vi "Determine Center of Gravity.vi"(0 "Input Intersections":T1(array[cluster])) -> (1 "CenterOfGravity X":dbl, 2 "CenterOfGravity Y":dbl)   [LabVIEW 2014, in "Position.lvclass"]
uses:
  Position.lvclass
  <vilib>/Analysis/NI_AALBase.lvlib
panel:
  out "y no":i32
  out "x no":i32
  out "x no":i32
  out "y no":i32
  # "This VI determines the center of gravity from a surface area.\nNotation: (x, y)"
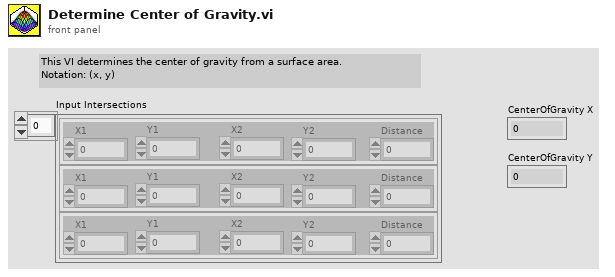
[diagram p1: front panel]
types:
  T1 = cluster{"X1":dbl, "Y1":dbl, "X2":dbl, "Y2":dbl, "Distance":dbl}[]
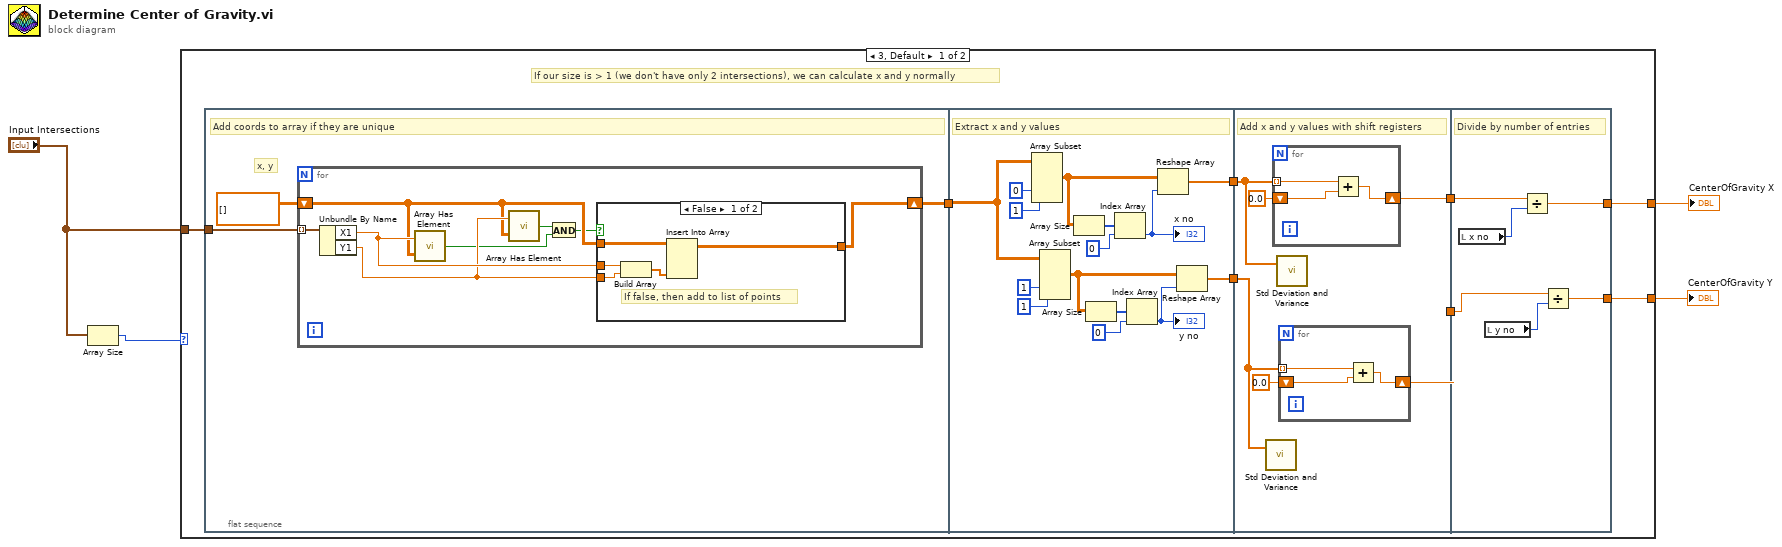
[diagram p0: block diagram]
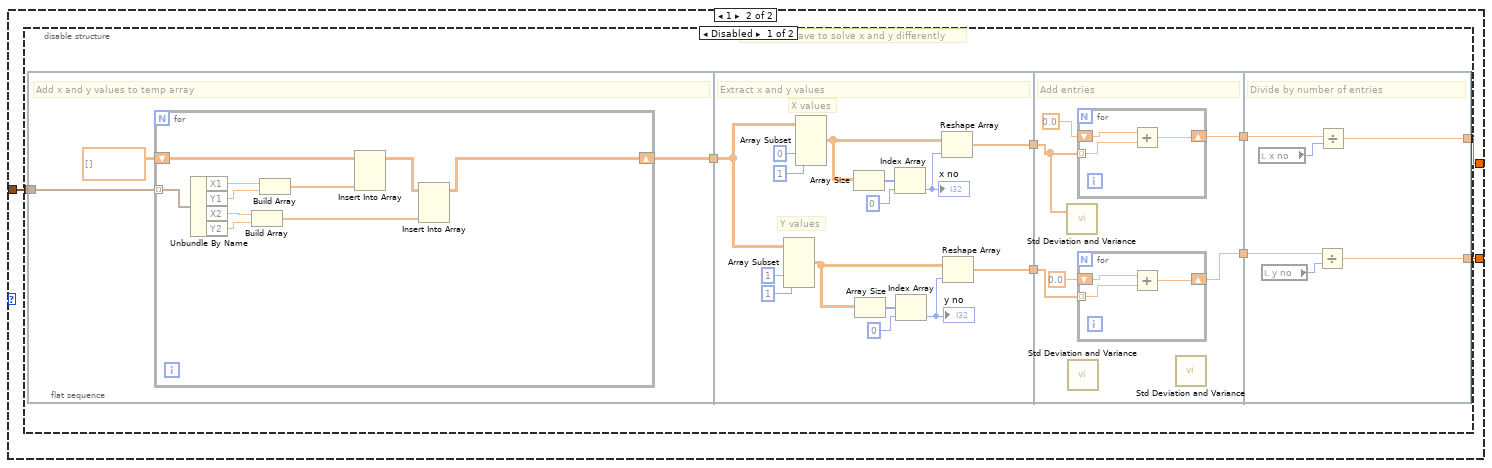
[diagram p3: hidden frame]
diagram:
  n1 = Array Size(array="Input Intersections") -> (size(s)=w1:i32)
  n2 = case shown="3, Default" w1 {
    tunnel: "Input Intersections" -> [w7 w65]
    tunnel: [w6 w63] -> w3
    tunnel: [w5 w64] -> w2
    frame 3, Default {
      # "If our size is > 1 (we don't have only 2 intersections), we can calculate x and y normally"
      n3 = flat-sequence {
        tunnel: w7 -> [w15]
        tunnel: [w14] -> w12
        tunnel: [w40] -> w11
        tunnel: [w39] -> w10
        tunnel: w12 -> [w30]
        tunnel: w11 -> [w46]
        tunnel: w10 -> [w45]
        tunnel: [w48] -> w9
        tunnel: [w47] -> w8
        tunnel: w9 -> [w61]
        tunnel: w8 -> [w60]
        tunnel: [w58] -> w6
        tunnel: [w57] -> w5
        frame #0 {
          # "x, y"
          # "Add coords to array if they are unique"
          n4 = for {
            tunnel: w15 -> [w23] mode=indexing
            shift-right: [w22] -> w14
            shift-left: dbl[][] [] -> [w19]
            n5 = Unbundle By Name(w23) -> ("X1"=w21:dbl, "Y1"=w20:dbl)
            n6 = call "Array Has Element.vi"("Array"=w19, "Element"=w21) -> ("Array has element?"=w17:bool)
            n7 = call "Array Has Element.vi"("Array"=w19, "Element"=w20) -> ("Array has element?"=w18:bool)
            n8 = And(x=w18, y=w17) -> (x .and. y?=w16:bool)
            n9 = case shown="False" w16 {
              tunnel: w21 -> [w27 _]
              tunnel: w20 -> [w26 _]
              tunnel: w19 -> [w28 w29]
              tunnel: [w24 w29] -> w22
              frame False {
                # "If false, then add to list of points"
                n10 = Build Array(w27, w26) -> (w25:dbl[])
                n11 = Insert Into Array(array=w28, new element=w25) -> (w24:dbl[][])  [unwired: 2 in]
              }
              frame True {
                # "If true, then don't add to list of points"
              }
            }
          }
        }
        frame #1 {
          # "Extract x and y values"
          n12 = Array Subset(array=w30, index (col)=0 ("index"), length (col)=1 ("length")) -> (w34:dbl[][])  [unwired: 2 in]
          n13 = Array Subset(array=w30, index (col)=1 ("index"), length (col)=1 ("length")) -> (w38:dbl[][])  [unwired: 2 in]
          n14 = Array Size(array=w34) -> (size(s)=w33:i32[])
          n15 = Array Size(array=w38) -> (size(s)=w37:i32[])
          n16 = Index Array(array=w33, index=0) -> (element=w31:i32)
          "x no" <- w31
          n17 = Index Array(array=w37, index=0) -> (element=w35:i32)
          "y no" <- w35
          n18 = Reshape Array(w34, w31) -> (w40:dbl[])
          n19 = Reshape Array(w38, w35) -> (w39:dbl[])
        }
        frame #2 {
          # "Add x and y values with shift registers"
          n20 = call <vilib>:"Std Deviation and Variance.vi"("X"=w45) -> ()  [unwired: 1 in, 3 out]
          n21 = for {
            tunnel: w46 -> [w54] mode=indexing
            shift-right: [w55] -> w48
            shift-left: 0.0 -> [w56]
            n22 = Add(x=w54, y=w56) -> (x+y=w55:dbl)
          }
          n23 = call <vilib>:"Std Deviation and Variance.vi"("X"=w46) -> ()  [unwired: 1 in, 3 out]
          n24 = for {
            tunnel: w45 -> [w53] mode=indexing
            shift-right: [w51] -> w47
            shift-left: 0.0 -> [w52]
            n25 = Add(x=w53, y=w52) -> (x+y=w51:dbl)
          }
        }
        frame #3 {
          # "Divide by number of entries"
          n26 = local read "x no"() -> (w62:i32)
          n27 = local read "y no"() -> (w59:i32)
          n28 = Divide(x=w61, y=w62) -> (x/y=w58:dbl)
          n29 = Divide(x=w60, y=w59) -> (x/y=w57:dbl)
        }
      }
    }
    frame 1 {
      n30 = disable-structure shown="Disabled" {
        disable-tunnel: w65 -> [w68 _]
        disable-tunnel: [w67 _] -> w64
        disable-tunnel: [w66 _] -> w63
        frame Disabled {
          # "Else, we'll have to solve x and y differently"
          n31 = flat-sequence {
            tunnel: w68 -> [w76]
            tunnel: [w74] -> w73
            tunnel: w73 -> [w99]
            tunnel: [w90] -> w72
            tunnel: [w87] -> w71
            tunnel: w72 -> [w102]
            tunnel: w71 -> [w106]
            tunnel: [w104] -> w70
            tunnel: [w103] -> w69
            tunnel: w70 -> [w119]
            tunnel: w69 -> [w117]
            tunnel: [w115] -> w67
            tunnel: [w114] -> w66
            frame #0 {
              # "Add x and y values to temp array"
              n32 = for {
                tunnel: w76 -> [w86] mode=indexing
                shift-right: [w78] -> w74
                shift-left: dbl[][] [] -> [w83]
                n33 = Unbundle By Name(w86) -> ("X1"=w85:dbl, "Y1"=w84:dbl, "X2"=w81:dbl, "Y2"=w80:dbl)
                n34 = Build Array(w81, w80) -> (w77:dbl[])
                n35 = Build Array(w85, w84) -> (w82:dbl[])
                n36 = Insert Into Array(array=w83, new element=w82) -> (w79:dbl[][])  [unwired: 2 in]
                n37 = Insert Into Array(array=w79, new element=w77) -> (w78:dbl[][])  [unwired: 2 in]
              }
            }
            frame #1 {
              # "Y values"
              # "X values"
              # "Extract x and y values"
              n38 = Array Subset(array=w99, index (col)=1 ("index"), length (col)=1 ("length")) -> (w89:dbl[][])  [unwired: 2 in]
              n39 = Array Subset(array=w99, index (col)=0 ("index"), length (col)=1 ("length")) -> (w92:dbl[][])  [unwired: 2 in]
              n40 = Array Size(array=w92) -> (size(s)=w95:i32[])
              n41 = Array Size(array=w89) -> (size(s)=w93:i32[])
              n42 = Index Array(array=w95, index=0) -> (element=w91:i32)
              "x no" <- w91
              n43 = Index Array(array=w93, index=0) -> (element=w88:i32)
              "y no" <- w88
              n44 = Reshape Array(w92, w91) -> (w90:dbl[])
              n45 = Reshape Array(w89, w88) -> (w87:dbl[])
            }
            frame #2 {
              # "Add entries"
              n46 = call <vilib>:"Std Deviation and Variance.vi"("X"=w102) -> ()  [unwired: 1 in, 3 out]
              n47 = call <vilib>:"Std Deviation and Variance.vi"() -> ()  [unwired: 2 in, 3 out]
              n48 = for {
                shift-right: [w111] -> w104
                shift-left: 0.0 -> [w113]
                tunnel: w102 -> [w112] mode=indexing
                n49 = Add(x=w113, y=w112) -> (x+y=w111:dbl)
              }
              n50 = for {
                shift-right: [w108] -> w103
                shift-left: 0.0 -> [w110]
                tunnel: w106 -> [w109] mode=indexing
                n51 = Add(x=w110, y=w109) -> (x+y=w108:dbl)
              }
              n52 = call <vilib>:"Std Deviation and Variance.vi"() -> ()  [unwired: 2 in, 3 out]
            }
            frame #3 {
              # "Divide by number of entries"
              n53 = local read "x no"() -> (w118:i32)
              n54 = local read "y no"() -> (w116:i32)
              n55 = Divide(x=w117, y=w116) -> (x/y=w115:dbl)
              n56 = Divide(x=w119, y=w118) -> (x/y=w114:dbl)
            }
          }
        }
        frame Enabled {
        }
      }
    }
  }
  "CenterOfGravity X" <- w3
  "CenterOfGravity Y" <- w2
